vi "Nested Malleable VIs - Lesson 3.vi"() -> ()   [LabVIEW 2023]
doc: "Lesson 3 discusses the concept of functor classes in more detail."
uses:
  Equal Via Regular Expression Functor/Equal Via Regular Expression Functor.lvclass
  Equal With Epsilon Functor/Equal With Epsilon Functor.lvclass
  Equal With Epsilon Functor/Equal With Epsilon Functor.lvclass/Equal With Epsilon Functor.ctl
  e4f9fbd4-fd76-40a4-bfcb-de5f69e1e77e.vi
  b4e98a28-dbdd-4fc2-834f-ccdb5c20f924.vi
  e4f9fbd4-fd76-40a4-bfcb-de5f69e1e77e.vi/5f008cf9-0835-42d5-ab12-715ade7a221f.vi
  b4e98a28-dbdd-4fc2-834f-ccdb5c20f924.vi/5f008cf9-0835-42d5-ab12-715ade7a221f.vi
  e4f9fbd4-fd76-40a4-bfcb-de5f69e1e77e.vi/5f008cf9-0835-42d5-ab12-715ade7a221f.vi/4a937600-749b-4ff4-8f55-34e6a7c3203b.vi
  b4e98a28-dbdd-4fc2-834f-ccdb5c20f924.vi/5f008cf9-0835-42d5-ab12-715ade7a221f.vi/4a937600-749b-4ff4-8f55-34e6a7c3203b.vi
  Equal Via Regular Expression Functor/Equals.vi
  Equal With Epsilon Functor/Equals.vi
panel:
  out "index of element 2":i32
  out "index of element 1":i32
  # "Overview: This lesson discusses functors, seen in the previous lesson, in more detail.\n\nInstructions: \n1. Open the block diagram of this VI. Review the lessons presented there.\n2. Run the VI to see the results. \n3. Once you have finished reviewing this VI, open the next lesson VI in the Malleable VIs - Nested Malleable VIs example project."
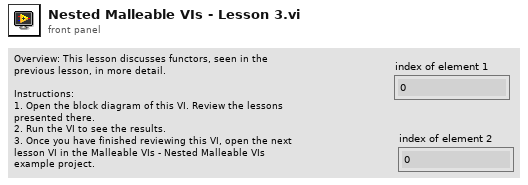
[diagram p1: front panel]
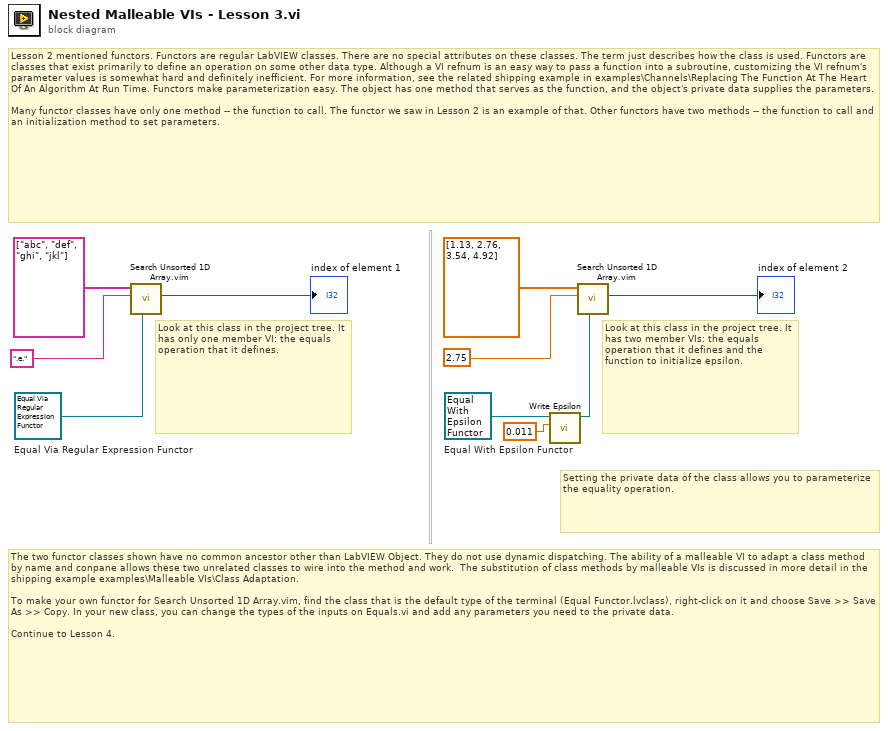
[diagram p0: block diagram]
diagram:
  w4 = refnum<class "Equal With Epsilon Functor.lvclass"> refnum  # Equal With Epsilon Functor
  w7 = refnum<class "Equal Via Regular Expression Functor.lvclass"> refnum  # Equal Via Regular Expression Functor
  # "The two functor classes shown have no common ancestor other than LabVIEW Object. They do not use dynamic dispatching. The ability of a malleable VI to adapt a class method by name and conpane allows these two unrelated classes to wire into the method and work.  The substitution of class methods by malleable VIs is discussed in more detail in the shipping example examples\\Malleable VIs\\Class Adaptation.\n\nTo make your own functor for Search Unsorted 1D Array.vim, find the class that is the default type of the terminal (Equal Functor.lvclass), right-click on it and choose Save >> Save As >> Copy. In your new class, you can change the types of the inputs on Equals.vi and add any parameters you need to the private data.\n\nContinue to Lesson 4."
  # "Setting the private data of the class allows you to parameterize the equality operation."
  # "Look at this class in the project tree. It has two member VIs: the equals operation that it defines and the function to initialize epsilon."
  # "Look at this class in the project tree. It has only one member VI: the equals operation that it defines."
  # "Lesson 2 mentioned functors. Functors are regular LabVIEW classes. There are no special attributes on these classes. The term just describes how the class is used. Functors are classes that exist primarily to define an operation on some other data type. Although a VI refnum is an easy way to pass a function into a subroutine, customizing the VI refnum's parameter values is somewhat hard and definitely inefficient. For more information, see the related shipping example in examples\\Channels\\Replacing The Function At The Heart Of An Algorithm At Run Time. Functors make parameterization easy. The object has one method that serves as the function, and the object's private data supplies the parameters.\n\nMany functor classes have only one method -- the function to call. The functor we saw in Lesson 2 is an example of that. Other functors have two methods -- the function to call and an initialization method to set parameters."
  n1 = call "Search Unsorted 1D Array.vim"("equals function (built-in =)"=w7, "element"=".e.", "unsorted 1D array"=string[] ["abc", "def", "ghi", "jkl"] ("1D array")) -> ("index of element"=→"index of element 1":i32)  [unwired: 8 in]
  n2 = call "Write Epsilon.vi"("epsilon"=0.011, "Equal With Epsilon Functor in"=w4) -> ("Equal With Epsilon Functor out"=w2:refnum<class "Equal With Epsilon Functor.lvclass">)  [unwired: 9 in]
  n3 = call "Search Unsorted 1D Array.vim"("equals function (built-in =)"=w2, "element"=2.75 ("epsilon"), "unsorted 1D array"=dbl[] [1.13, 2.76, 3.54, 4.92] ("1D array")) -> ("index of element"=→"index of element 2":i32)  [unwired: 8 in]
